vi "get No of Samples.vi"(8 "error in (no error)":errorcluster, 11 "Automation in":refnum<class "NMR Data.lvclass">) -> (0 "error out":errorcluster, 2 "Number of samples taken":i32, 3 "Automation out":refnum<class "NMR Data.lvclass">)   [LabVIEW 2019, in "NMR Data.lvclass"]
uses:
  NMR Data.lvclass
  NMR Data.lvclass/NMR Data.ctl
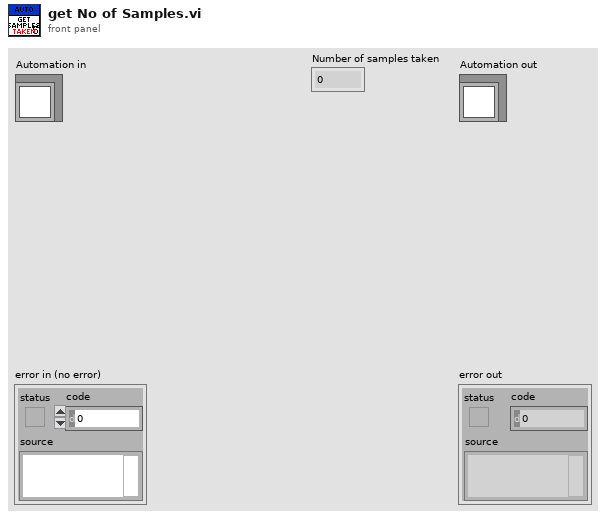
[diagram p1: front panel]
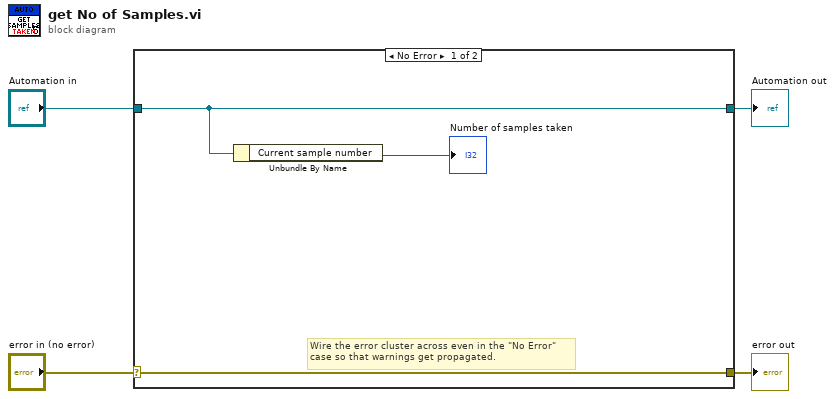
[diagram p0: block diagram]
diagram:
  n1 = case shown="No Error" "error in (no error)" {
    selector: "error in (no error)" -> [w7 w9]
    tunnel: [w7 w9] -> w3
    tunnel: [w6 w8] -> w1
    tunnel: "Automation in" -> [w6 w8]
    frame No Error {
      # "Wire the error cluster across even in the \"No Error\"\ncase so that warnings get propagated."
      n2 = Unbundle By Name(w6) -> ("Current sample number"=→"Number of samples taken":i32)
    }
    frame Error {
    }
  }
  "error out" <- w3
  "Automation out" <- w1
